vi "test.vi"() -> ()   [LabVIEW 2018]
uses:
  ti2_lightPath.ctl
  ti2_filterPos.ctl
  ti2lv.lvlib
panel:
  in  "Enable Joystick":bool
  in  "y Position Set (um)":dbl
  in  "x Position Set (um)":dbl
  out "y Position (um)":dbl
  out "x Position (um)":dbl
  out "pUserOutParam":i32[](array[numeric])
  in  "Filter Position Set":T1=1 items=["1"=1, "2"=2, "3"=3, "4"=4, "5"=5, "6"=6]
  out "Filter Position":T1=1 items=["1"=1, "2"=2, "3"=3, "4"=4, "5"=5, "6"=6]
  in  "Light Path Set":T2=1 items=["Eyepieces"=1, "Right"=2, "Bottom"=3, "Left"=4]
  in  "z Position Set (um)":dbl
  out "Light Path":T2=1 items=["Eyepieces"=1, "Right"=2, "Bottom"=3, "Left"=4]
  out "z Position (um)":dbl
  in  "Stop":bool
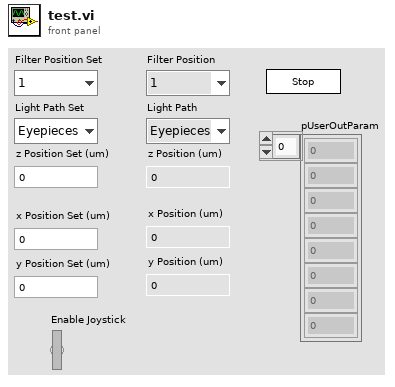
[diagram p1: front panel]
types:
  T1 = typedef "ti2lv.lvlib/ti2_filterPos.ctl" = u16
  T2 = typedef "ti2lv.lvlib/ti2_lightPath.ctl" = i32
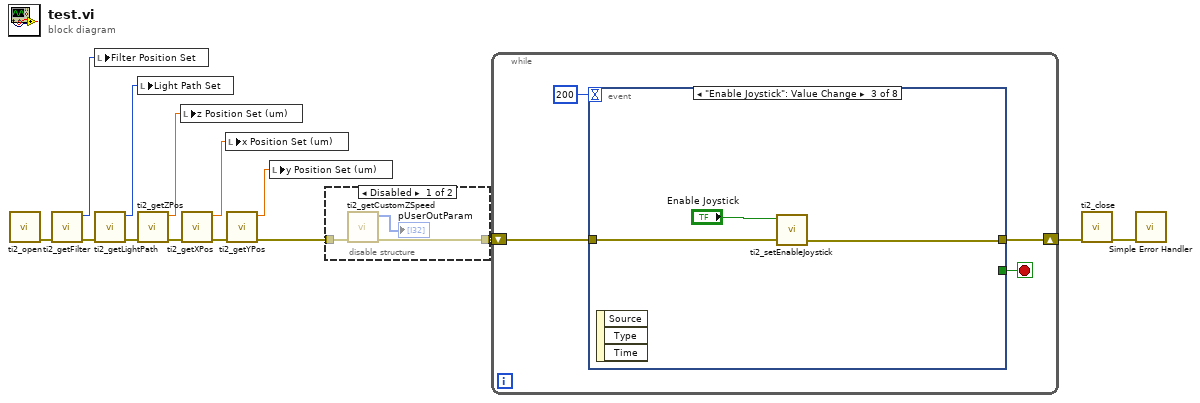
[diagram p0: block diagram]
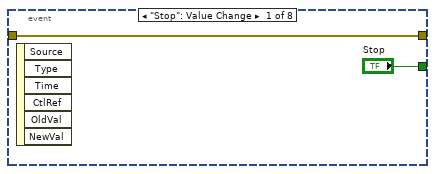
[diagram p3: hidden frame]
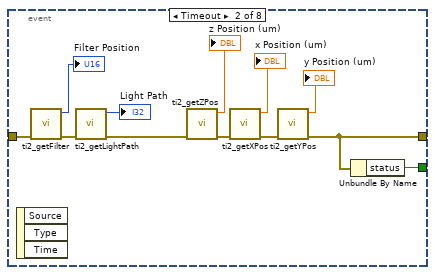
[diagram p4: hidden frame]
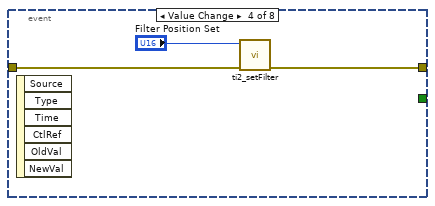
[diagram p5: hidden frame]
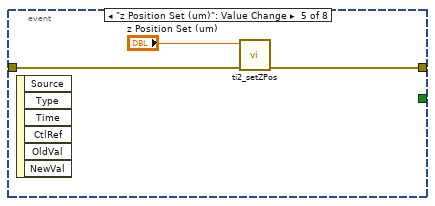
[diagram p6: hidden frame]
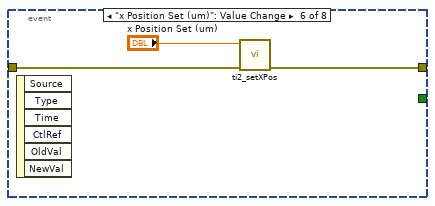
[diagram p7: hidden frame]
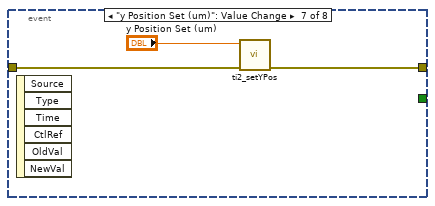
[diagram p8: hidden frame]
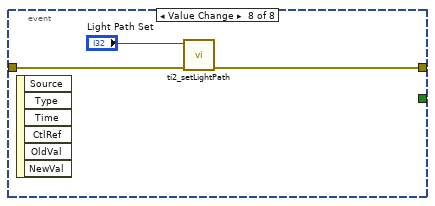
[diagram p9: hidden frame]
diagram:
  n1 = call "ti2_open.vi"() -> ("error out"=w12:errorcluster)  [unwired: 11 in]
  n2 = call "ti2_getFilter.vi"("error in (no error)"=w12) -> ("error out"=w13:errorcluster, "Filter Position"=w11:T1)  [unwired: 9 in]
  n3 = local write "Filter Position Set"(w11) -> ()
  n4 = call "ti2_getLightPath.vi"("error in (no error)"=w13) -> ("error out"=w14:errorcluster, "Light Path"=w10:T2)  [unwired: 9 in]
  n5 = local write "Light Path Set"(w10) -> ()
  n6 = call "ti2_getZPos.vi"("error in (no error)"=w14) -> ("error out"=w7:errorcluster, "z Position (um)"=w9:dbl)  [unwired: 9 in]
  n7 = local write "z Position Set (um)"(w9) -> ()
  n8 = call "ti2_getXPos.vi"("error in (no error)"=w7) -> ("error out"=w5:errorcluster, "x Position (um)"=w6:dbl)  [unwired: 9 in]
  n9 = local write "x Position Set (um)"(w6) -> ()
  n10 = call "ti2_getYPos.vi"("error in (no error)"=w5) -> ("error out"=w1:errorcluster, "y Position (um)"=w4:dbl)  [unwired: 9 in]
  n11 = local write "y Position Set (um)"(w4) -> ()
  n12 = disable-structure shown="Disabled" {
    disable-tunnel: [w17 _] -> w8
    disable-tunnel: w1 -> [w15 _]
    frame Disabled {
      n13 = call "ti2_getCustomZSpeed.vi"("error in (no error)"=w15) -> ("error out"=w17:errorcluster, "pUserOutParam"=→"pUserOutParam":i32[])  [unwired: 9 in]
    }
    frame Enabled {
    }
  }
  n14 = while {
    shift-right: [w19] -> w2
    shift-left: w8 -> [w20]
    stop <- w21 stop-if-true
    n15 = event shown="[2] \"Enable Joystick\": Value Change" {
      selector: _ -> [_ _ _ _ _ _ _ _]
      dyn-events: _ -> [_ _ _ _ _ _ _ _]
      timeout: 200 -> [_ _ _ _ _ _ _ _]
      tunnel: ["Stop" w25 _ _ _ _ _ _] -> w21
      tunnel: w20 -> [w22 w35 w38 w41 w44 w46 w49 w53]
      tunnel: [w22 w24 w37 w40 w42 w45 w48 w52] -> w19
      event "Stop": Value Change {
        n16 = event-data() -> ()  [unwired: 1 in, 6 out]
      }
      event Timeout {
        n17 = event-data() -> ()  [unwired: 1 in, 3 out]
        n18 = call "ti2_getFilter.vi"("error in (no error)"=w35) -> ("error out"=w34:errorcluster, "Filter Position"=→"Filter Position":T1)  [unwired: 9 in]
        n19 = call "ti2_getLightPath.vi"("error in (no error)"=w34) -> ("error out"=w33:errorcluster, "Light Path"=→"Light Path":T2)  [unwired: 9 in]
        n20 = call "ti2_getZPos.vi"("error in (no error)"=w33) -> ("error out"=w29:errorcluster, "z Position (um)"=→"z Position (um)":dbl)  [unwired: 9 in]
        n21 = call "ti2_getXPos.vi"("error in (no error)"=w29) -> ("error out"=w27:errorcluster, "x Position (um)"=→"x Position (um)":dbl)  [unwired: 9 in]
        n22 = call "ti2_getYPos.vi"("error in (no error)"=w27) -> ("error out"=w24:errorcluster, "y Position (um)"=→"y Position (um)":dbl)  [unwired: 9 in]
        n23 = Unbundle By Name(w24) -> ("status"=w25:bool)
      }
      event "Enable Joystick": Value Change {
        n24 = event-data() -> ()  [unwired: 1 in, 3 out]
        n25 = call "ti2_setEnableJoystick.vi"("error in (no error)"=w38, "value"="Enable Joystick") -> ("error out"=w37:errorcluster)  [unwired: 9 in]
      }
      event Value Change {
        n26 = event-data() -> ()  [unwired: 1 in, 6 out]
        n27 = call "ti2_setFilter.vi"("error in (no error)"=w41, "Filter Position"="Filter Position Set") -> ("error out"=w40:errorcluster)  [unwired: 9 in]
      }
      event "z Position Set (um)": Value Change {
        n28 = event-data() -> ()  [unwired: 1 in, 6 out]
        n29 = call "ti2_setZPos.vi"("error in (no error)"=w44, "z Position (um)"="z Position Set (um)") -> ("error out"=w42:errorcluster)  [unwired: 9 in]
      }
      event "x Position Set (um)": Value Change {
        n30 = event-data() -> ()  [unwired: 1 in, 6 out]
        n31 = call "ti2_setXPos.vi"("error in (no error)"=w46, "x Position (um)"="x Position Set (um)") -> ("error out"=w45:errorcluster)  [unwired: 9 in]
      }
      event "y Position Set (um)": Value Change {
        n32 = event-data() -> ()  [unwired: 1 in, 6 out]
        n33 = call "ti2_setYPos.vi"("error in (no error)"=w49, "y Position (um)"="y Position Set (um)") -> ("error out"=w48:errorcluster)  [unwired: 9 in]
      }
      event Value Change {
        n34 = event-data() -> ()  [unwired: 1 in, 6 out]
        n35 = call "ti2_setLightPath.vi"("error in (no error)"=w53, "Light Path"="Light Path Set") -> ("error out"=w52:errorcluster)  [unwired: 9 in]
      }
    }
  }
  n36 = call "ti2_close.vi"("error in (no error)"=w2) -> ("error out"=w3:errorcluster)  [unwired: 10 in]
  n37 = call <vilib>:"Simple Error Handler.vi"("error in (no error)"=w3) -> ()  [unwired: 4 in, 5 out]
